vi "sum_function(SubVI).vi"(0 "10":bool, 1 "20":bool, 2 "50":bool, 3 "1":bool, 4 "2":bool, 5 "5":bool, 6 "Sum IN":dbl) -> (7 "Sum OUT":dbl)   [LabVIEW 2013]
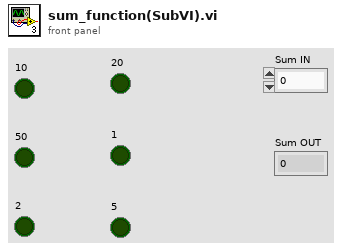
[diagram p1: front panel]
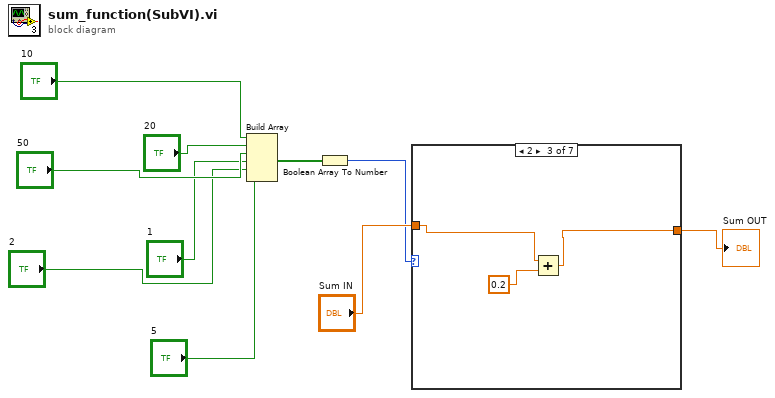
[diagram p0: block diagram]
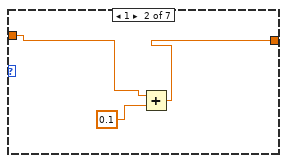
[diagram p3: hidden frame]
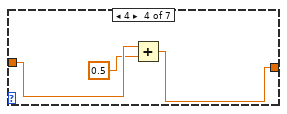
[diagram p4: hidden frame]
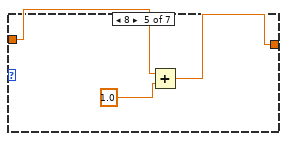
[diagram p5: hidden frame]
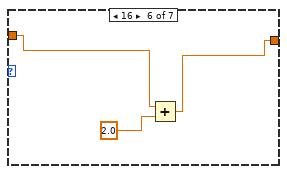
[diagram p6: hidden frame]
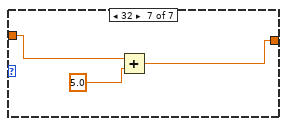
[diagram p7: hidden frame]
diagram:
  n1 = Build Array("10", "20", "50", "1", "2", "5") -> (w10:bool[])
  n2 = Boolean Array To Number(Boolean array=w10) -> (number=w1:u32)
  n3 = case shown="2" w1 {
    tunnel: "Sum IN" -> [w11 w13 w15 w20 w22 w25 w28]
    tunnel: [w11 w12 w16 w19 w21 w24 w27] -> w2
    frame 0, Default {
    }
    frame 1 {
      n4 = Add(x=w13, y=0.1) -> (x+y=w12:dbl)
    }
    frame 2 {
      n5 = Add(x=w15, y=0.2) -> (x+y=w16:dbl)
    }
    frame 4 {
      n6 = Add(x=w20, y=0.5) -> (x+y=w19:dbl)
    }
    frame 8 {
      n7 = Add(x=w22, y=1.0) -> (x+y=w21:dbl)
    }
    frame 16 {
      n8 = Add(x=w25, y=2.0) -> (x+y=w24:dbl)
    }
    frame 32 {
      n9 = Add(x=w28, y=5.0) -> (x+y=w27:dbl)
    }
  }
  "Sum OUT" <- w2
